vi "Read DAQmx Synthesizer Configuration.vi"(8 "error in (no error)":errorcluster, 11 "DAQmx Synthesizer in":refnum<class "DAQmx Synthesizer.lvclass">) -> (0 "error out":errorcluster, 2 "Configuration":T1={"Channel names"=[], "Output channels"="0:1", "Waveform file"=path "", "Offset"=1.0, "Scale"=0.5, "Ranges"=[10.0], "Post-trigger delay"=0.01, "Post-trigger duration"=0.1, "Rate"=1000000.0, "Re-name channels"=[], "Active channels"="0:1", "External\nclock"=FALSE} {"Rate" format="%#_8pHz"; "Post-trigger duration" format="%#_6ps"; "Post-trigger delay" format="%#_6ps"; "Ranges" format="%#_6pV"}, 3 "DAQmx Synthesizer out":refnum<class "DAQmx Synthesizer.lvclass">)   [LabVIEW 2021, in "DAQmx Synthesizer.lvclass"]
uses:
  DAQmx Synthesizer.lvclass
  C:/GitHub/NHMFL_Core/Libraries/Instruments/Instrument Driver/Instrument Driver.lvclass
  DAQmx Synthesizer Configuration.ctl
  DAQmx Synthesizer.lvclass/DAQmx Synthesizer.ctl
panel:
  # "Pulse config"
  # "Waveform generation config"
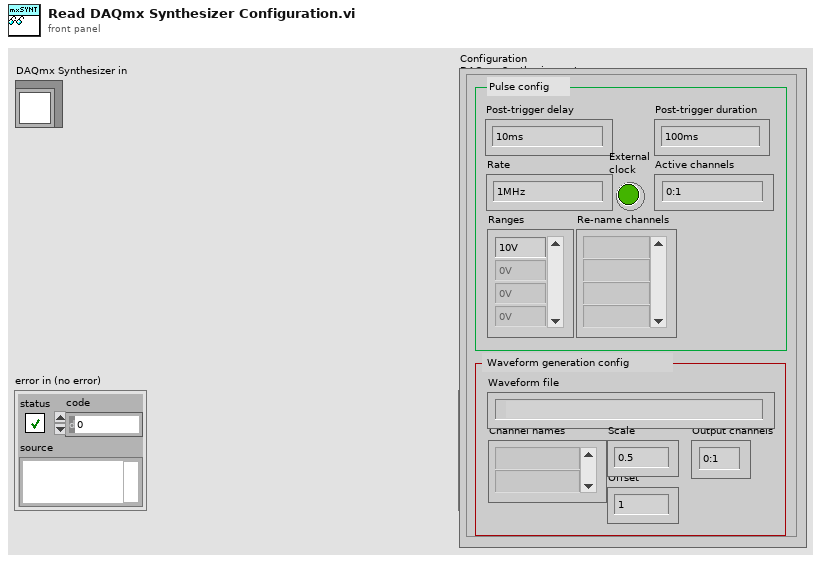
[diagram p1: front panel]
types:
  T1 = typedef "DAQmx Synthesizer Configuration.ctl" = cluster{"Channel names":string[], "Output channels":string, "Waveform file":path, "Offset":dbl, "Scale":dbl, "Ranges":dbl[], "Post-trigger delay":dbl, "Post-trigger duration":dbl, "Rate":dbl, "Re-name channels":string[], "Active channels":string, "External\nclock":bool}
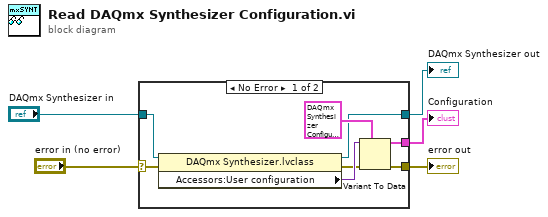
[diagram p0: block diagram]
diagram:
  n1 = case shown="No Error" "error in (no error)" {
    selector: "error in (no error)" -> [w13 w14]
    tunnel: [w7 w14] -> w4
    tunnel: [w10 w15] -> w2
    tunnel: "DAQmx Synthesizer in" -> [w11 w15]
    tunnel: [w6 _] -> w1
    frame No Error {
      n2 = property class="DAQmx Synthesizer.lvclass"(reference=w11, error in=w13) -> (reference out=w10:refnum<class "DAQmx Synthesizer.lvclass">, error out=w8:errorcluster, "Accessors:User configuration"=w9:variant)
      n3 = Variant To Data(error in=w8, type=T1 {"Channel names"=[], "Output channels"="0:1", "Waveform file"=path "", "Offset"=1.0, "Scale"=0.5, "Ranges"=[10.0], "Post-trigger delay"=0.01, "Post-trigger duration"=0.1, "Rate"=1000000.0, "Re-name channels"=[], "Active channels"="0:1", "External\nclock"=FALSE} ("Configuration"), Variant=w9) -> (data=w6:T1, error out=w7:errorcluster)
    }
    frame Error {
    }
  }
  "error out" <- w4
  "DAQmx Synthesizer out" <- w2
  "Configuration" <- w1
